vi "Deserialize Connection Info.vi"(7 "Field Delimiter (::)":string="::", 8 "error in (no error)":errorcluster, 11 "Connection Info String":string) -> (0 "error out":errorcluster, 3 "Deserialized Connection Info":T1={"VISA Resource"="", "Address"=1} {"Address" min=1})   [LabVIEW 2020, in "plugin_flodx_pressure.lvlib" / "plugin.lvlib" / "Instrument Manager.lvlib"]
doc: "Deserializes a connection info string. By default, it deserializes a string in the format \"<visa_resource>::<pump_address>\"."
uses:
  Instrument Manager.lvlib
  Connection Info.ctl
panel:
  out "homogenized string":string
  # "Debug"
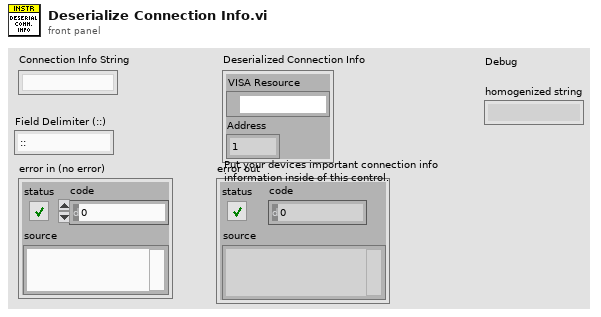
[diagram p1: front panel]
types:
  T1 = typedef "plugin_flodx_pressure.lvlib/plugin.lvlib/Instrument Manager.lvlib/Connection Info.ctl" = cluster{"VISA Resource":refnum<visa-resource-name>, "Address":u8}
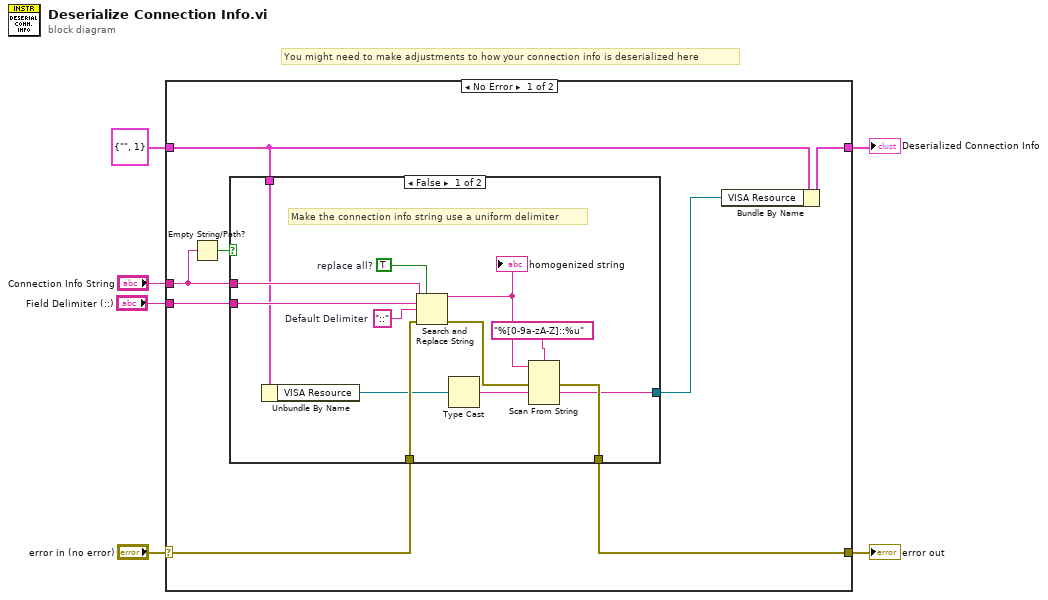
[diagram p0: block diagram]
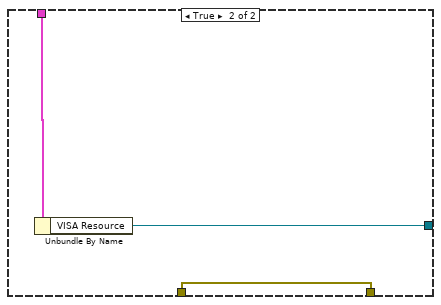
[diagram p2: hidden frame]
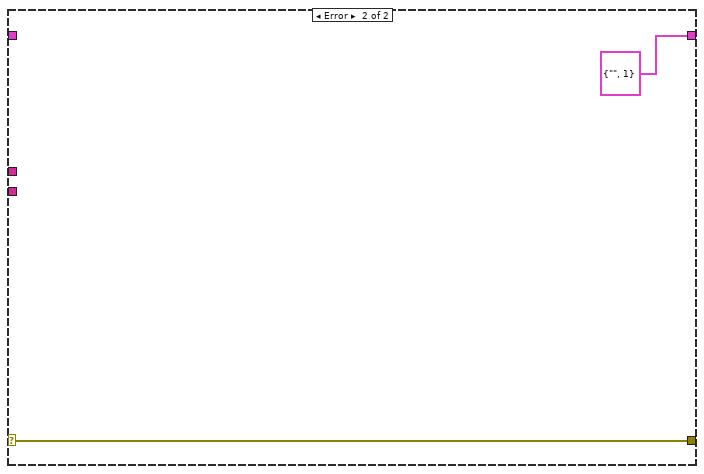
[diagram p3: hidden frame]
diagram:
  # "You might need to make adjustments to how your connection info is deserialized here"
  n1 = case shown="No Error" "error in (no error)" {
    selector: "error in (no error)" -> [w13 w32]
    tunnel: [w14 w32] -> w5
    tunnel: "Field Delimiter (::)" -> [w12 _]
    tunnel: [w11 T1 {"VISA Resource"="", "Address"=1} ("Deserialized Connection Info")] -> w3
    tunnel: "Connection Info String" -> [w7 _]
    tunnel: T1 {"VISA Resource"="", "Address"=1} ("Deserialized Connection Info") -> [w9 _]
    frame No Error {
      n2 = Empty String/Path?(string/path=w7) -> (empty?=w8:bool)
      n3 = case shown="False" w8 {
        tunnel: [w27 w28] -> w14
        tunnel: w13 -> [w26 w28]
        tunnel: w7 -> [w21 _]
        tunnel: w12 -> [w20 _]
        tunnel: [w17 w29] -> w10
        tunnel: w9 -> [w15 w30]
        frame False {
          w24 = TRUE  # replace all?
          w19 = "::"  # Default Delimiter
          # "Make the connection info string use a uniform delimiter"
          n4 = Unbundle By Name(w15) -> ("VISA Resource"=w23:refnum<visa-resource-name>)
          n5 = Search and Replace String(replace all?=w24, input string=w21, search string=w20, replace string=w19, error in=w26) -> (result string=w16:string, error out=w25:errorcluster)  [unwired: 3 in, 2 out]
          "homogenized string" <- w16
          n6 = Type Cast(x=w23) -> (*(type *) &x=w18:string)  [unwired: 1 in]
          n7 = Scan From String(format string="%[0-9a-zA-Z]::%u" ("Format String"), input string=w16, error in=w25, default 1=w18) -> (error out=w27:errorcluster, output 1=w17:string)  [unwired: 3 in, 2 out]
        }
        frame True {
          n8 = Unbundle By Name(w30) -> ("VISA Resource"=w29:refnum<visa-resource-name>)
        }
      }
      n9 = Bundle By Name(cluster=w9, "VISA Resource"=w10) -> (w11:T1)
    }
    frame Error {
    }
  }
  "error out" <- w5
  "Deserialized Connection Info" <- w3
